vi "File Folder Filter.vi"(8 "error in":errorcluster, 10 "pattern":string[](array[string]), 11 "Selection":path[](array[path])) -> (0 "error out":errorcluster, 3 "All Files in Dir":path[](array[path]))   [LabVIEW 2019, in "SimpleDependencyInspector.lvlib"]
uses:
  SimpleDependencyInspector.lvlib
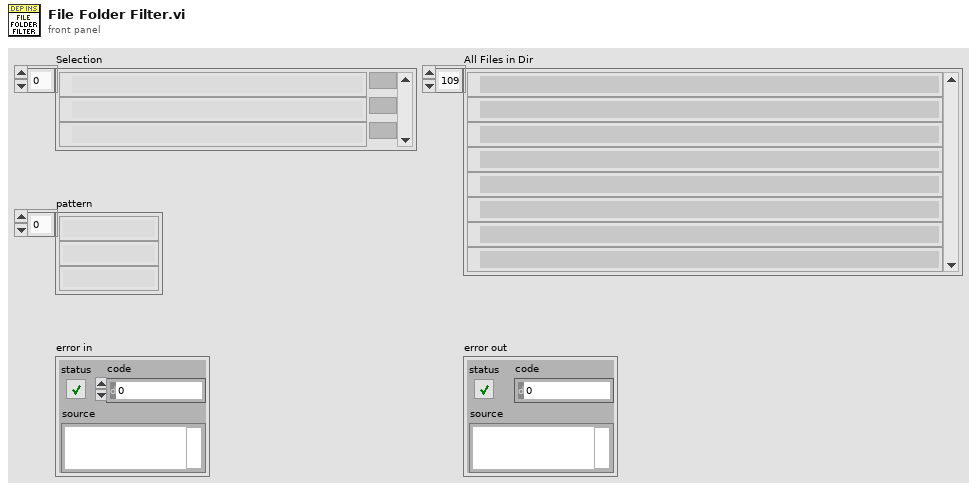
[diagram p1: front panel]
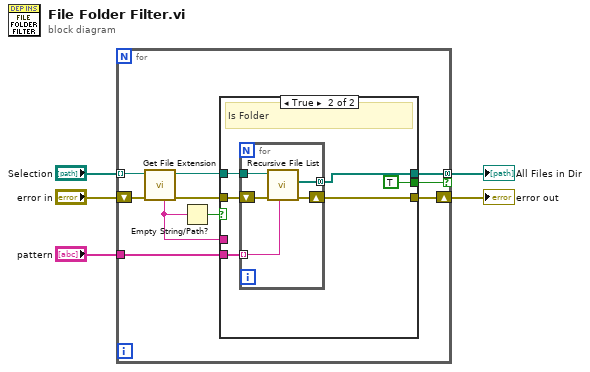
[diagram p0: block diagram]
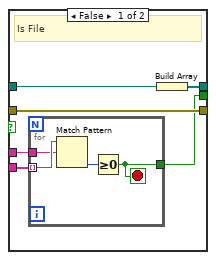
[diagram p2: hidden frame]
diagram:
  n1 = for {
    tunnel: "Selection" -> [w10] mode=indexing
    tunnel: [w12] -> w2 mode=concatenating if=w6
    shift-right: [w15] -> w5
    shift-left: "error in" -> [w14]
    tunnel: "pattern" -> [w11]
    n2 = call <vilib>:"Get File Extension.vi"("error in (no error)"=w14, "file"=w10) -> ("error out"=w13:errorcluster, "dup file"=w9:path, "unmodified file extension"=w7:string)  [unwired: 5 in, 2 out]
    n3 = Empty String/Path?(string/path=w7) -> (empty?=w8:bool)
    n4 = case shown="True" w8 {
      tunnel: [w21 w31] -> w15
      tunnel: [w19 w29] -> w12
      tunnel: w11 -> [w18 w28]
      tunnel: w13 -> [w21 w30]
      tunnel: w9 -> [w20 w27]
      tunnel: w7 -> [w17 _]
      tunnel: [w16 TRUE] -> w6
      frame False {
        # "Is File"
        n5 = for {
          tunnel: w18 -> [w25] mode=indexing
          tunnel: w17 -> [w24]
          tunnel: [w22] -> w16
          stop <- w22 stop-if-true
          n6 = Match Pattern(string=w25, regular expression=w24) -> (offset past match=w23:i32)  [unwired: 1 in, 3 out]
          n7 = Greater Or Equal To 0?(x=w23) -> (x >= 0?=w22:bool)
        }
        n8 = Build Array(w20) -> (w19:path[])
      }
      frame True {
        # "Is Folder"
        n9 = for {
          tunnel: w27 -> [w34]
          tunnel: [w33] -> w29 mode=concatenating
          shift-right: [w35] -> w31
          shift-left: w30 -> [w36]
          tunnel: w28 -> [w32] mode=indexing
          n10 = call <vilib>:"Recursive File List.vi"("pattern"=w32, "error in (no error)"=w36, "Folder Path"=w34) -> ("error out"=w35:errorcluster, "All Files in Dir"=w33:path[])  [unwired: 4 in, 3 out]
        }
      }
    }
  }
  "All Files in Dir" <- w2
  "error out" <- w5
